vi "Main.vi"() -> ()   [LabVIEW 2015]
doc: "This Continuous Measurement sample project is based on the Queued Message Handler template.\n\nThe Event Handling Loop generates messages based on user interface actions.\n\nThe Message Handling Loop processes messages generated by the Event Handling Loop, or by other messages. There are also Acquisition and Logging message handling loop subVIs, and a chart updating loop."
uses:
  controls/Test Data.ctl
  controls/Tags.ctl
  controls/UI State.ctl
  controls/Flota.ctl
  support/Message Queue/Enqueue Message (Single).vi
  support/Message Queue/Enqueue Message (Array).vi
  <vilib>/Utility/error.llb/Error Cluster From Error Code.vi
  <vilib>/ErrorRing/Error Ring.xnode
  support/User Event - Stop/User Event - Stop.lvlib
  support/Message Queue/Message Queue.lvlib
panel:
  in  "Acq":T1
  in  "TAGs":T2
  out "Ultimo TEST":timestamp
  in  "Test":T3
  out "Reset del controlador":bool
  out "error":errorcluster
  in  "Developer commad":string
  out "Buffer Overflow":bool
  out "Buffer Underflow":bool
  in  "Calibration":bool
  out "Report":string
  in  "Exit":bool
  # "Opciones\n- Adquirir\n- STOP_WHD\n- Reset_Controlador"
  # "Misma función que introducir STOP_WHD\n en Developer command"
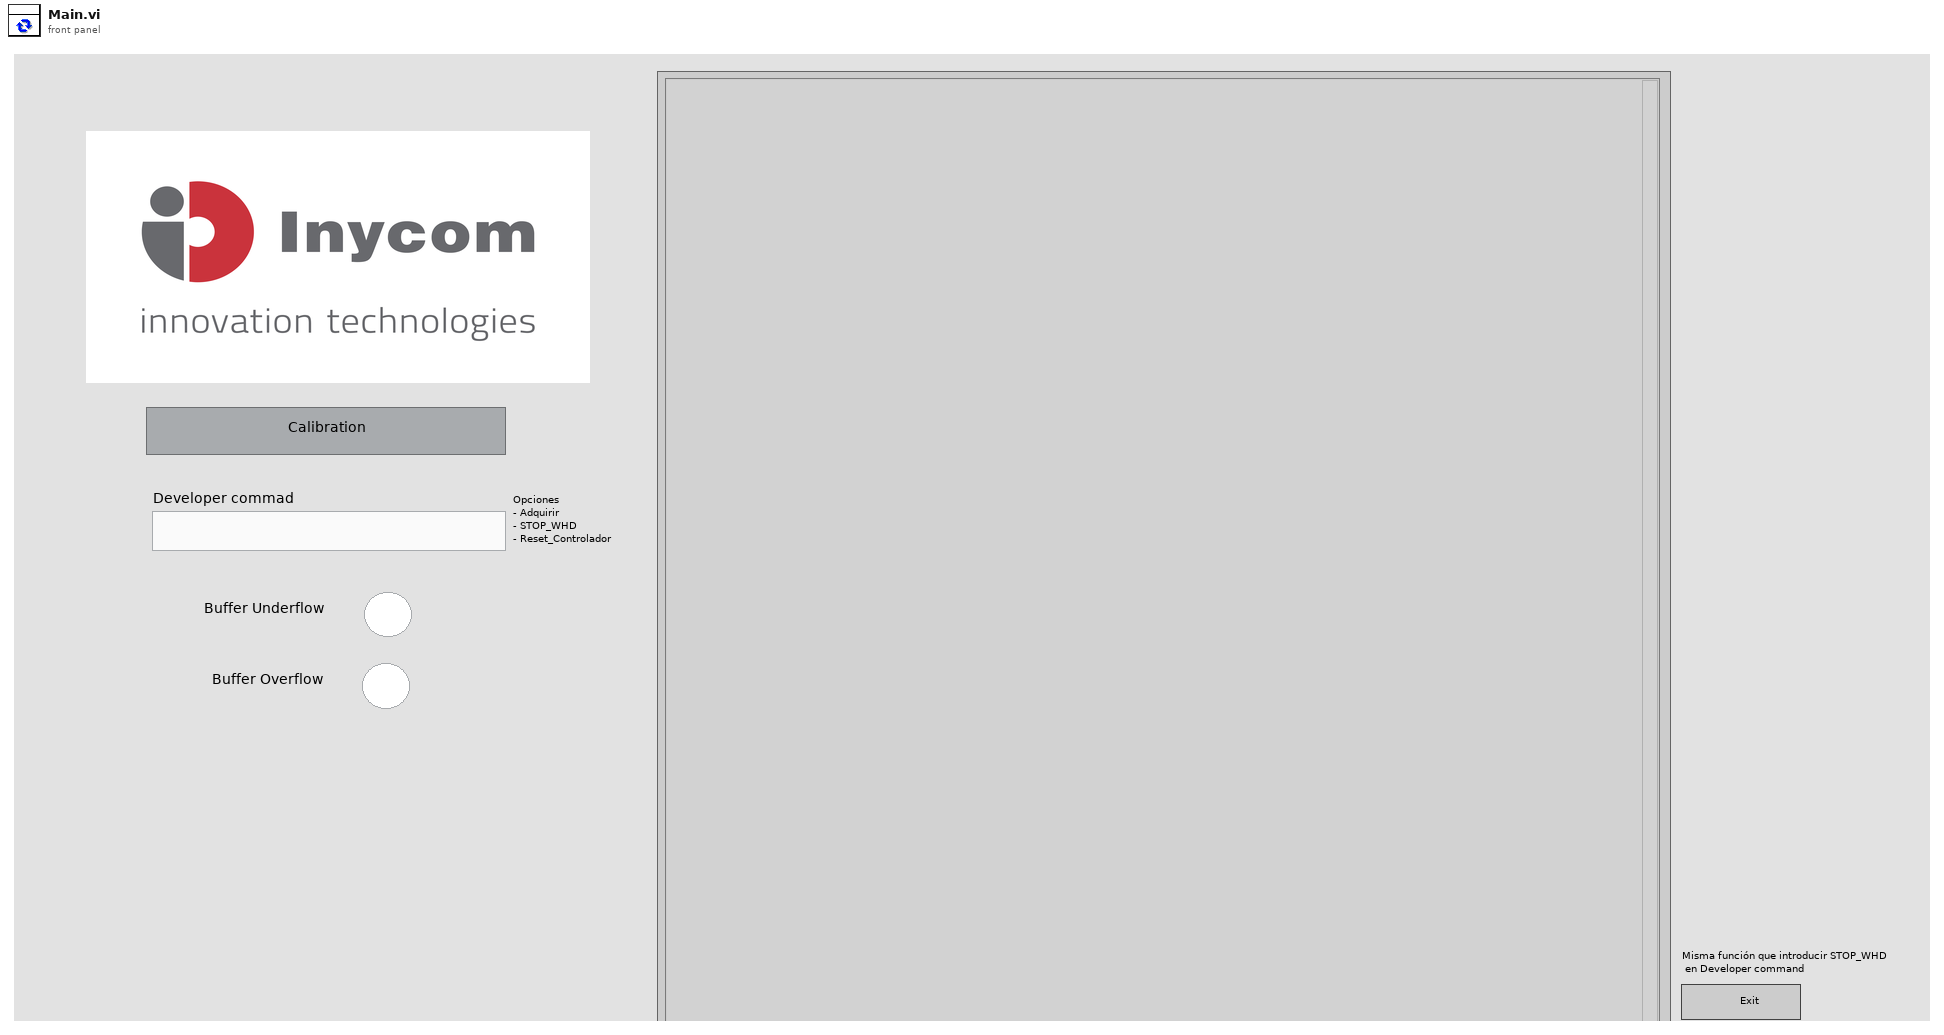
[diagram p1: front panel]
types:
  T1 = cluster{"FPGA error ":errorcluster, "data":dbl[], "Direccion 0?":bool, "File error ":errorcluster}
  T2 = typedef "Tags.ctl" = cluster{"TAGs":string[], "TAGs HEX":string[], "TAGs LR6":string[], "it-read-LR6":i32[], "it-LR6":i32}
  T3 = typedef "Test Data.ctl" = cluster{"DC OK":string, "Aviso temperatura":string, "Aviso no detección":string, "RuedaDetectada1?":bool, "RuedaDetectada2?":bool, "T fuera rango":bool, "Fallo Fotocelula":bool, "Timeout ruedas":bool, "Buffer Underflow":bool, "Buffer Overflow":bool, "Nº Ruedas 1":i32, "NºRuedas 2":i32, "Block Size":u32, "Time to Acquire Block (ms)":i32, "Ref file Data":refnum<file>[], "Number of elements":u32, "Tiempo de paso (s)":dbl}
  T4 = typedef "UI State.ctl" = enum16{"Idle", "Waiting_trigger", "Acquiring and Logging", "Calibration", "Waiting for Exit", "Waiting for Exit (Acq Stopped)", "Waiting for Exit (Log Stopped)", "Waiting for Stop", "Waiting for Stop (Acq Stopped)", "Waiting for Stop (Log Stopped)"}
  T5 = typedef "File paths.ctl" = cluster{"configuration":path, "confRFID":path, "LOG.txt":path, "Path LOG":path, "Path_data":path, "TAGS leidos":path, "configuracion flota":path, "flota":path, "Nombre de archivo":path[], "Folder calibration":path, "calibration log":path, "Reporting Procesamiento":path, "Error ejes":path, "Reporting Adquisición":path}
  T6 = cluster{"error IO":errorcluster, bool[], u32[], string[], dbl[]}
  T7 = typedef "Cfg_parameters.ctl" = cluster{"RFID NEM on?":bool, "RFID LR6 on?":bool, "Use Aura?":bool, "Leer config RFID NEM":bool, "Canal cero WS1?":bool, "Canal cero WS2 ":bool, "Digital?":bool, "Reset watchdog?":bool, "Able watchdog?":bool, "Borrar archivos\nadquisicion con error":bool, "AURA wheel test":bool, "Save calibration":bool, "Puerto RFID":u16, "Port LR6":u16, "timeout ms (60000)":i32, "bytes to read":i32, "DeviceAddress":u8, "IP RFID":string, "IP synchr":string, "LR6 IP address":string, "Parametros AuraWheel":string[], "Frecuencia de muestreo y módulo CRIO":T8, "Escaneos de la FIFO por canal":u32, "Frecuencia de muestreo (Hz)":dbl, "dt RMS":dbl, "Tiempo extra al detector de paso (s)":dbl, "Count(mSec)":u32, "Offset_rueda WS 1":fxp<+/-,24,-4>, "Offset_rueda WS 2":fxp<+/-,24,-4>, "Nº de acelerómetros":i32, "Nº inductivos":i32, "Max archivos":u32, "Bytes min libre":u32, "Bytes libre despues de borrar":u32, "Timeout ruedas":dbl, "Pattern amplitude (g)":dbl, "Pattern frequency (Hz)":dbl, "Tiempo de adquisicion\n":dbl, "Parámetros acelerómetros":dbl[], "Inicio pasada":timestamp, "Ultimo TEST":timestamp, "Report_AURA":string, "Temperatura (ºC)":dbl, "Direccion 0?":bool}
  T8 = typedef "nicrio_cRIO-9234_DataRatesRing2.ctl" = u8
  T9 = typedef "Message Queue.lvlib/All Message Queues.ctl" = cluster{"UI":refnum<queue>, "Acquisition and Logging":refnum<queue>, "RFID":refnum<queue>, "Processing":refnum<queue>, "Watchdog":refnum<queue>, "Calibration":refnum<queue>}
  T10 = typedef "Flota.ctl" = cluster{"Series_flota":string[], "Distancia de acelerómetros":dbl[], "Puntos medios de las ventanas":dbl[][], "Distancias generales":dbl[], "Tabla_flota":string[][]}
  T11 = cluster{"Distacias y medidas de dispositivos":bool, "Lectura_OK?":bool}
  T12 = cluster{"FPGA error ":errorcluster, "data":dbl[], "TAGs":string[], "Direccion 0?":bool}
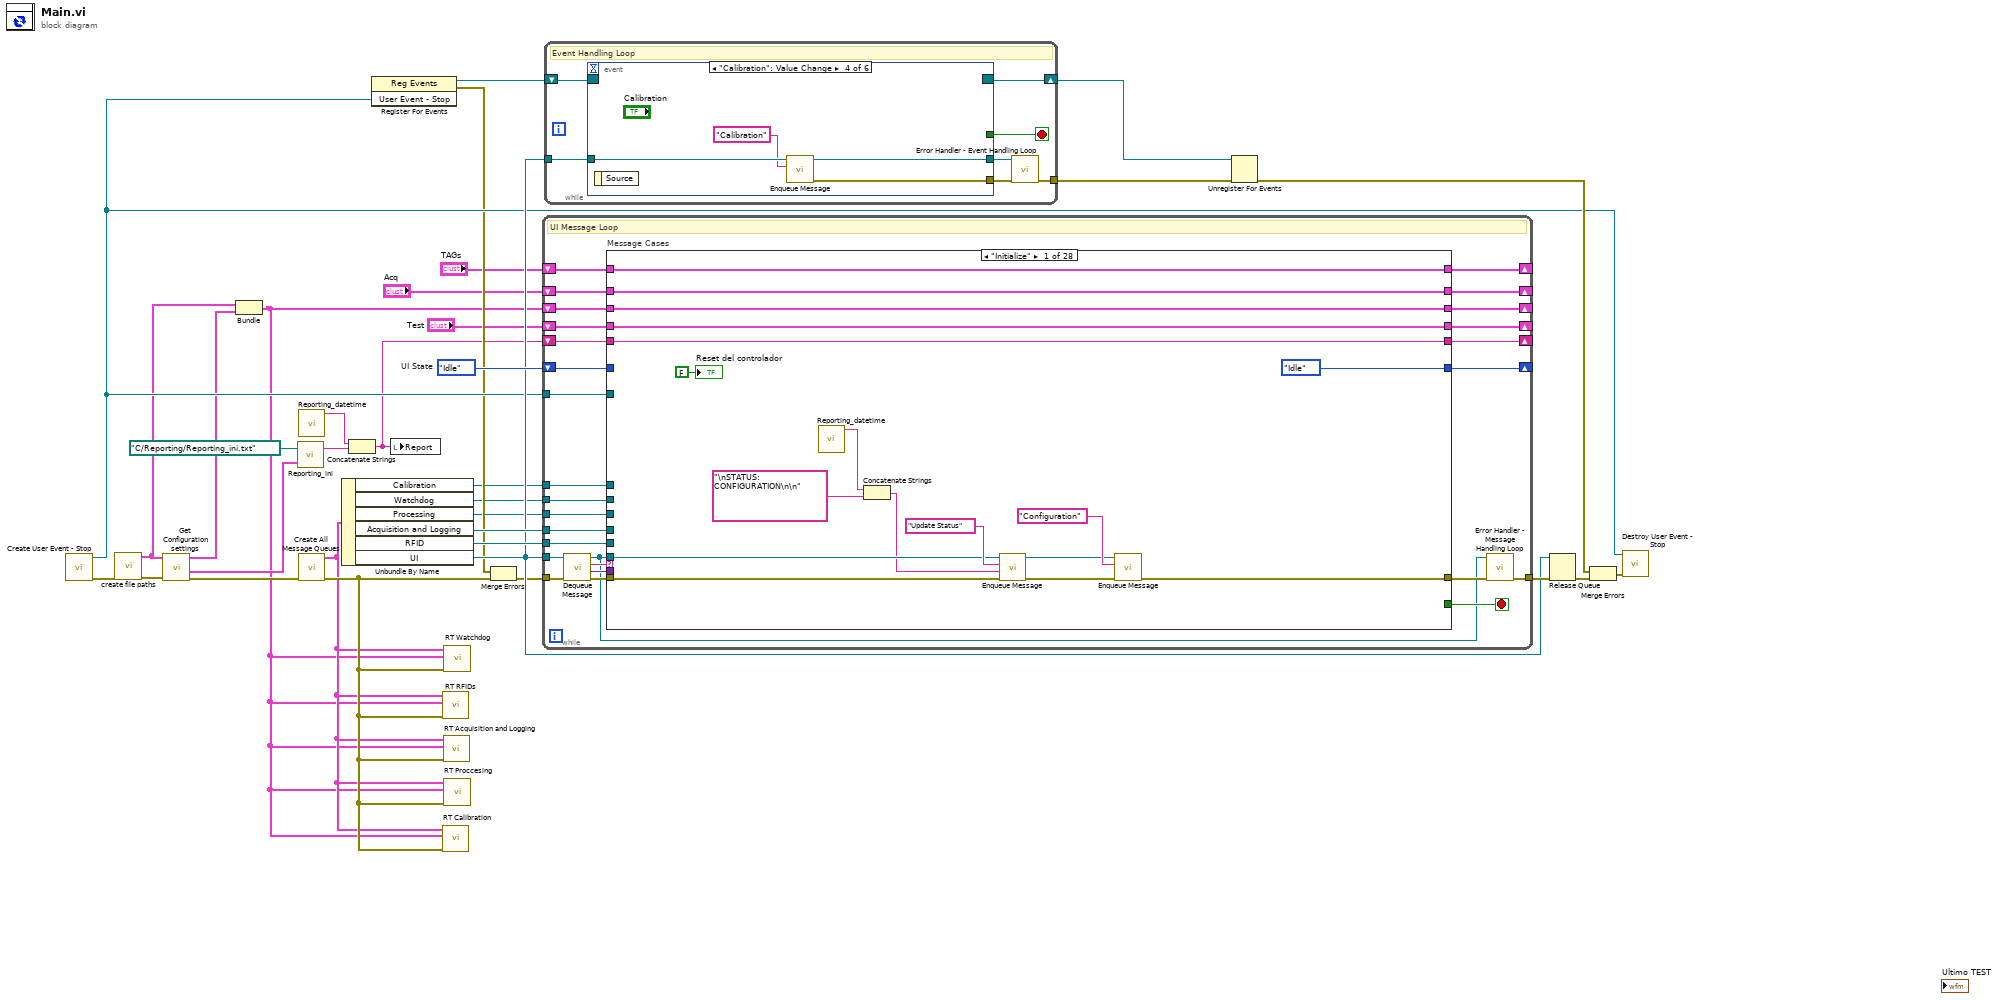
[diagram p0: block diagram]
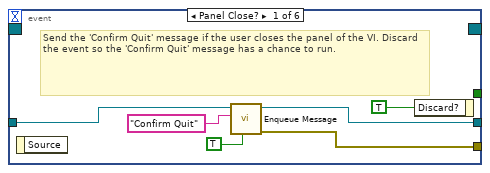
[diagram p2: hidden frame]
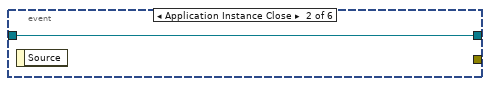
[diagram p3: hidden frame]
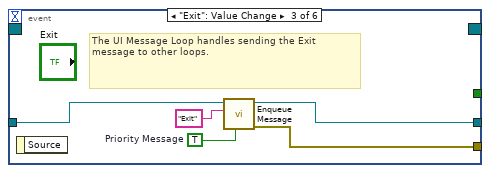
[diagram p4: hidden frame]
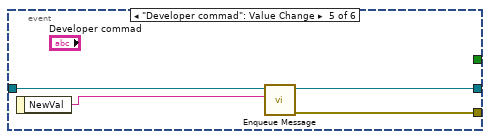
[diagram p5: hidden frame]
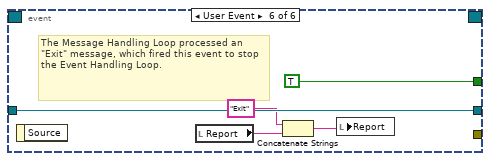
[diagram p6: hidden frame]
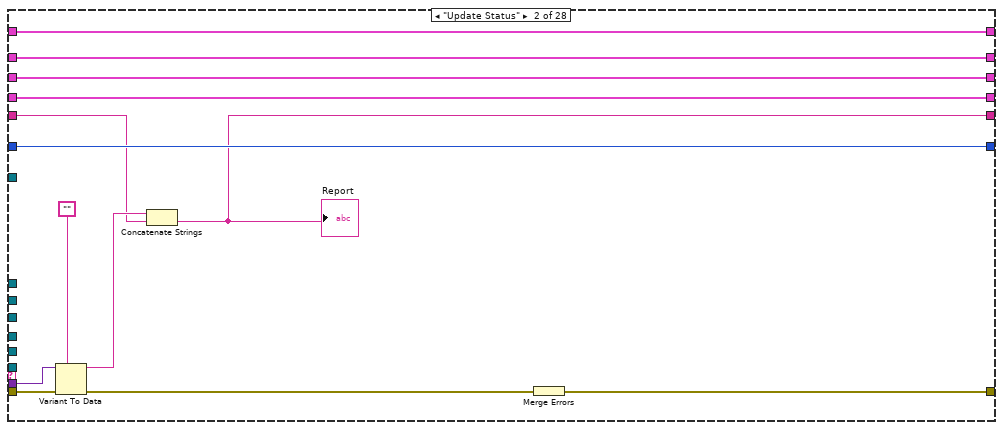
[diagram p7: hidden frame]
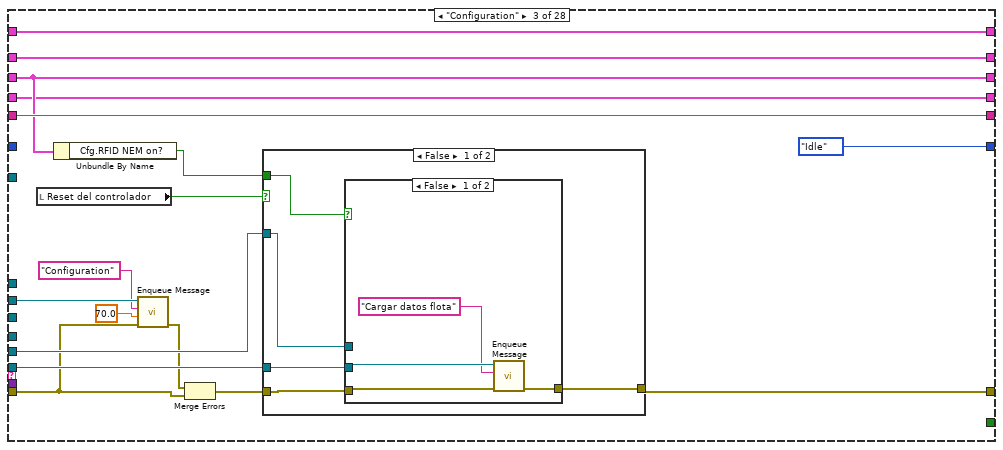
[diagram p8: hidden frame]
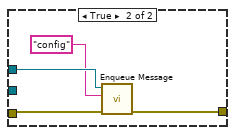
[diagram p9: hidden frame]
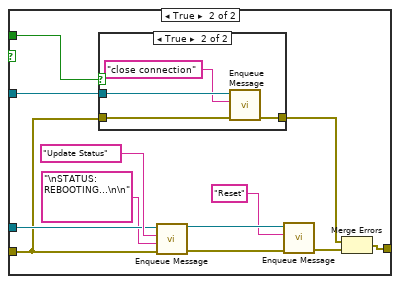
[diagram p10: hidden frame]
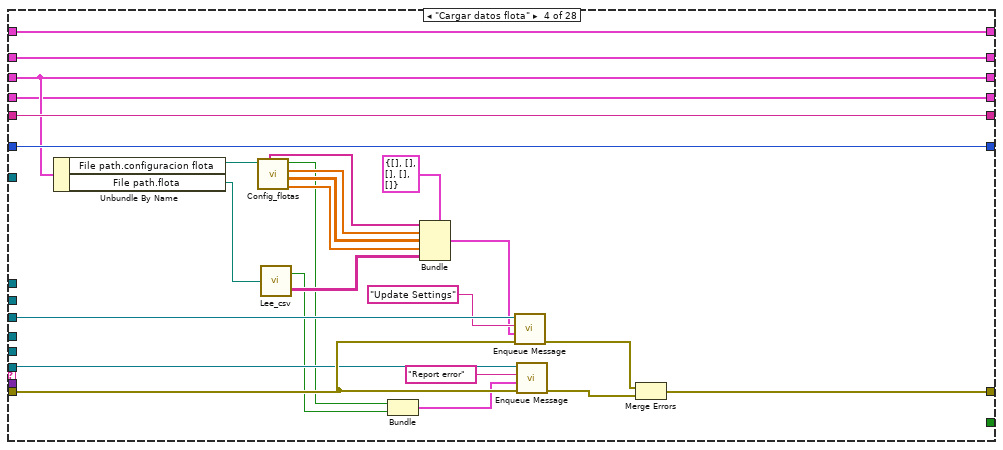
[diagram p12: hidden frame]
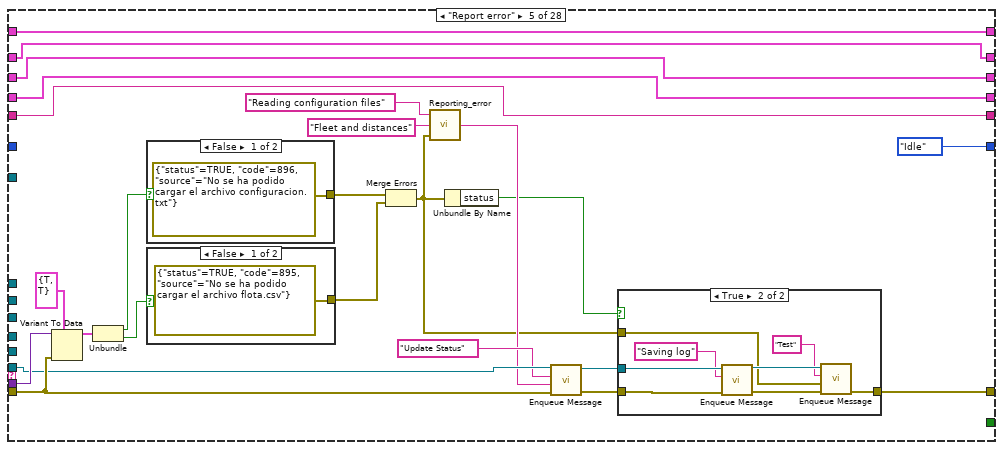
[diagram p13: hidden frame]
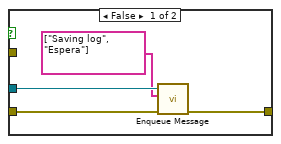
[diagram p14: hidden frame]
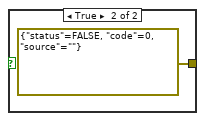
[diagram p15: hidden frame]
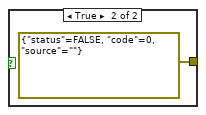
[diagram p16: hidden frame]
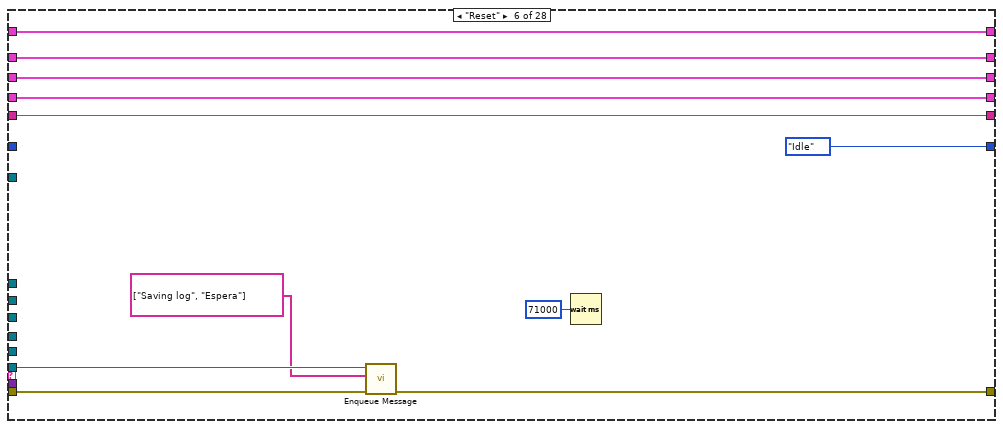
[diagram p17: hidden frame]
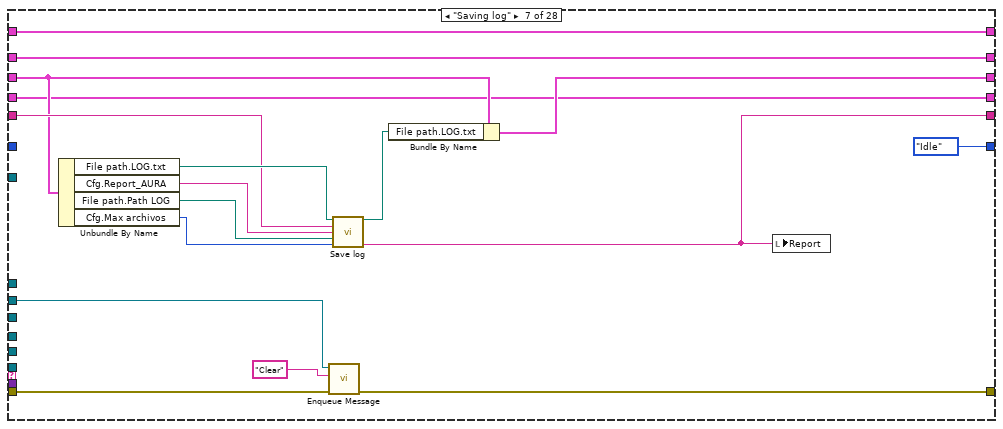
[diagram p18: hidden frame]
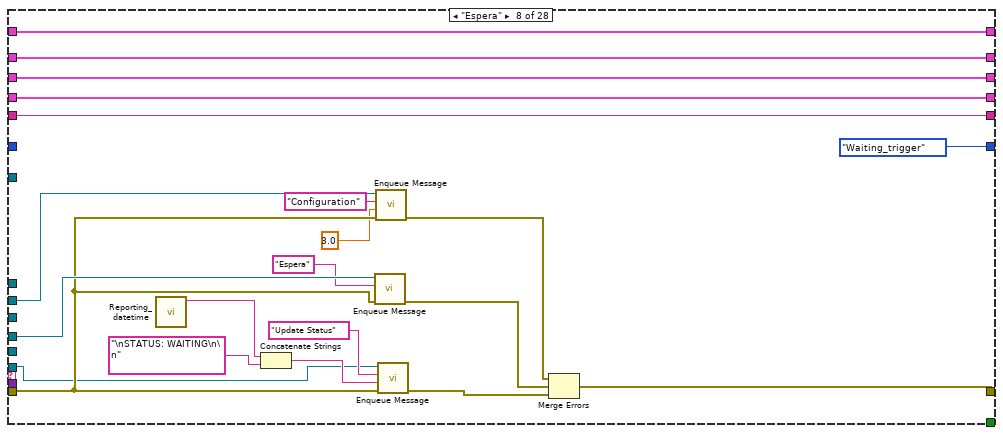
[diagram p19: hidden frame]
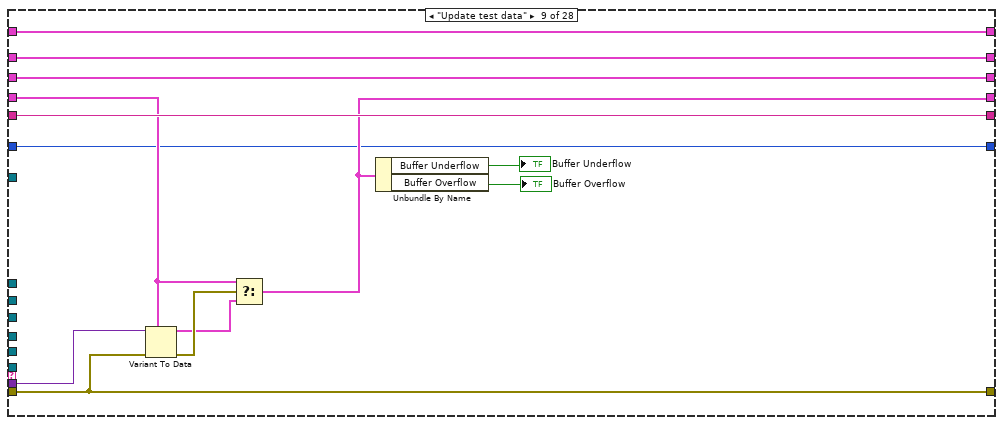
[diagram p20: hidden frame]
diagram:
  w27 = UI_State."Idle"  # UI State
  n1 = call "Create User Event - Stop.vi"() -> ("error out"=w13:errorcluster, "User Event - Stop"=w23:refnum<user-event>)  [unwired: 10 in]
  n2 = call "create file paths.vi"("error in"=w13) -> ("error out"=w12:errorcluster, "File path"=w11:T5)  [unwired: 9 in]
  n3 = call "Get Configuration settings.vi"("error in (no error)"=w12, "File path"=w11) -> ("error out"=w19:errorcluster, "output cluster"=w14:T6, "Cfg"=w10:T7)  [unwired: 5 in]
  n4 = Bundle("File path"=w11, "Cfg"=w10) -> (w2:cluster{"File path":T5, "Cfg ":T7})  [unwired: 1 in]
  n5 = call "Reporting_ini.vi"("Configuration cluster"=w14, "address repoting"=path "C:/Reporting/Reporting_ini.txt" ("file (use dialog)")) -> ("Reporting"=w17:string)  [unwired: 1 in]
  n6 = call "Reporting_datetime.vi"() -> ("String"=w16:string)  [unwired: 11 in]
  n7 = call "Create All Message Queues.vi"("error in (no error)"=w19) -> ("error out"=w4:errorcluster, "Message Queues out"=w3:T9)  [unwired: 9 in]
  n8 = Unbundle By Name(w3) -> ("Calibration"=w1:refnum<queue>, "Watchdog"=w8:refnum<queue>, "Processing"=w9:refnum<queue>, "Acquisition and Logging"=w29:refnum<queue>, "RFID"=w28:refnum<queue>, "UI"=w25:refnum<queue>)
  n9 = Concatenate Strings(w16, w17) -> (w15:string)
  n10 = register-events(w23) -> (reference out=w24:refnum<event-registration>, error out=w21:errorcluster)  [unwired: 2 in]
  n11 = local write "Report"(w15) -> ()
  n12 = call "RT RFIDs.vi"("error in (no error)"=w4, "info"=w2, "Message Queues in"=w3) -> ()  [unwired: 8 in, 1 out]
  n13 = call "RT Calibration.vi"("error in (no error)"=w4, "info"=w2, "Message Queues in"=w3) -> ()  [unwired: 8 in, 1 out]
  n14 = call "RT Acquisition and Logging.vi"("error in (no error)"=w4, "info"=w2, "Message Queues in"=w3) -> ()  [unwired: 8 in, 1 out]
  n15 = call "RT Watchdog.vi"("error in (no error)"=w4, "info"=w2, "Message Queues in"=w3) -> ()  [unwired: 8 in, 1 out]
  n16 = call "RT Proccesing.vi"("error in (no error)"=w4, "info"=w2, "Message Queues in"=w3) -> ()  [unwired: 8 in, 1 out]
  n17 = Merge Errors(w21, w4) -> (w22:errorcluster)
  n18 = while {
    tunnel: w25 -> [w54]
    tunnel: w23 -> [w59]
    shift-right: [w53] -> _
    shift-left: w2 -> [w52]
    tunnel: w29 -> [w51]
    tunnel: w28 -> [w50]
    shift-right: [w45] -> _
    shift-left: w27 -> [w46]
    tunnel: w22 -> [w58]
    tunnel: [w49] -> w33
    shift-right: [w43] -> _
    shift-left: w15 -> [w44]
    tunnel: w9 -> [w42]
    tunnel: w8 -> [w41]
    shift-right: [w39] -> _
    shift-left: "Test" -> [w40]
    shift-right: [w37] -> _
    shift-left: "TAGs" -> [w38]
    shift-right: [w35] -> _
    shift-left: "Acq" -> [w36]
    tunnel: w1 -> [w34]
    stop <- w60 stop-if-true
    # "UI Message Loop"
    n19 = call "Dequeue Message.vi"("error in (no error)"=w58, "Message Queue"=w54) -> ("error out"=w57:errorcluster, "Message Data"=w55:variant, "Message"=w56:string, "dup Message Queue"=w47:refnum<queue>)  [unwired: 6 in]
    n20 = case "Message Cases" shown="\"Initialize\"" w56 {
      selector: w56 -> [_ _ _ _ _ _ _ _ _ w271 _ _ _ _ _ _ _ _ _ _ _ _ _ _ _ _ _ w664]
      tunnel: w47 -> [w75 _ w102 w145 w175 w208 _ w236 _ _ w287 w300 _ w347 w379 w390 w438 w472 w491 w514 w541 w566 _ _ w609 _ _ _]
      tunnel: w57 -> [w74 w89 w96 w149 w176 w209 w222 w245 w260 w275 w286 w301 w320 w343 w365 w392 w439 w473 w492 w511 w527 w557 w582 w595 w608 w644 w658 _]
      tunnel: [w66 w90 w100 w148 w173 w210 w220 w244 w260 w275 w285 w299 w321 w339 w374 w391 w437 w471 w490 w508 w535 w559 w582 w597 w607 w648 w657 w663] -> w48
      tunnel: [_ _ _ _ _ _ _ _ _ _ _ _ _ _ _ _ _ _ _ _ _ _ _ _ _ TRUE _ _] -> w60
      tunnel: w55 -> [_ w88 _ _ w187 _ _ _ w261 _ _ _ _ _ w364 w402 w444 w479 w498 _ _ _ w580 w598 _ w642 _ _]
      tunnel: w59 -> [_ _ _ _ _ _ _ _ _ _ _ _ _ _ _ _ _ _ _ _ _ _ _ _ _ w649 _ _]
      tunnel: [w72 w83 w105 w161 w168 w214 w223 w252 w265 w274 w292 w303 w326 w350 w383 w387 w446 w482 w501 w519 w543 w576 w578 w601 w611 w647 w656 w666] -> w53
      tunnel: w52 -> [w72 w83 w105 w161 w168 w214 w225 w252 w265 w274 w292 w303 w326 w350 w383 w388 w446 w482 w501 w519 w543 w576 w579 w601 w611 w647 w656 w666]
      tunnel: w51 -> [_ _ _ _ _ _ _ w247 _ w272 _ w296 w319 _ _ _ w435 _ _ _ _ _ _ _ _ w640 _ _]
      tunnel: w50 -> [_ _ w101 _ _ _ _ _ _ _ _ _ _ w348 _ _ _ _ _ _ _ _ _ _ _ w646 _ _]
      tunnel: w46 -> [_ w85 _ w162 _ _ _ _ w253 w270 w290 w298 w324 _ _ _ _ w469 w488 _ _ w571 w585 w596 w610 _ w655 w665]
      tunnel: [UI_State."Idle" ("UI State") w85 UI_State."Idle" ("UI State") w162 UI_State."Idle" ("UI State") UI_State."Idle" ("UI State") UI_State."Idle" ("UI State") UI_State."Waiting_trigger" ("UI State") w253 w269 w290 w297 w323 UI_State."Acquiring and Logging" ("UI State") UI_State."Idle" ("UI State") UI_State."Idle" ("UI State") UI_State."Idle" ("UI State") UI_State."Waiting for Stop (Acq Stopped)" ("UI State") UI_State."Waiting for Stop (Acq Stopped)" ("UI State") UI_State."Idle" ("UI State") UI_State."Idle" ("UI State") w571 w585 w596 w606 UI_State."Idle" ("UI State") w655 w665] -> w45
      tunnel: w44 -> [w73 w81 w106 w163 w178 w211 w229 w237 w264 w273 w291 w302 w325 w335 w367 w393 w433 w477 w494 w525 w546 w572 w586 w594 w605 w641 w654 w662]
      tunnel: [w73 w84 w106 w163 w178 w211 w215 w237 w264 w273 w291 w302 w325 w335 w367 w393 w433 w477 w494 w525 w546 w572 w586 w594 w605 w641 w654 w662] -> w43
      tunnel: w42 -> [_ _ _ w152 _ _ _ _ _ _ _ _ _ _ _ _ _ _ _ _ _ w558 _ _ _ w639 _ _]
      tunnel: w41 -> [_ _ w99 _ _ _ w221 w246 _ _ _ _ _ w344 w375 w384 _ _ _ _ w534 w563 _ _ _ w638 _ _]
      tunnel: w40 -> [w63 w80 w93 w140 w169 w206 w218 w234 w259 w268 w283 w295 w322 w336 w368 w389 w434 w478 w495 w526 w542 w573 w587 w592 w604 w636 w653 w661]
      tunnel: [w63 w80 w93 w140 w169 w206 w218 w234 w258 w268 w283 w295 w322 w336 w368 w389 w434 w478 w495 w526 w542 w573 w587 w592 w604 w636 w653 w661] -> w39
      tunnel: w38 -> [w62 w79 w92 w139 w167 w205 w217 w233 w255 w267 w282 w294 w318 w338 w361 w386 w431 w476 w497 w522 w544 w575 w589 w591 w603 w635 w652 w660]
      tunnel: [w62 w79 w92 w139 w167 w205 w217 w233 w255 w267 w282 w294 w318 w338 w361 w386 w431 w476 w496 w522 w544 w575 w589 w591 w603 w635 w652 w660] -> w37
      tunnel: w36 -> [w61 w78 w91 w138 w166 w204 w216 w232 w254 w266 w281 w293 w317 w337 w360 w385 w430 w475 w493 w523 w532 w574 w588 w590 w602 w634 w651 w659]
      tunnel: [w61 w78 w91 w138 w166 w204 w216 w232 w254 w266 w281 w293 w317 w337 w360 w385 w430 w474 w493 w523 w532 w574 w588 w590 w602 w634 w651 w659] -> w35
      tunnel: w34 -> [_ _ _ _ _ _ _ _ _ _ _ _ _ _ _ _ _ _ _ _ _ _ _ _ _ w633 _ _]
      frame "Initialize" {
        # "Initialize - Get configuration settings, then message the UI to initialize, and broadcast the settings to the other message loops."
        n21 = call "Reporting_datetime.vi"() -> ("String"=w70:string)  [unwired: 11 in]
        n22 = Concatenate Strings(w70, "\nSTATUS: CONFIGURATION\n\n") -> (w69:string)
        n23 = call-poly "Enqueue Message.vi"("error in (no error)"=w74, "Message Data"=w69, "Message"="Update Status", "Message Queue"=w75) -> ("error out"=w67:errorcluster, "dup Message Queue"=w65:refnum<queue>)  [unwired: 6 in]
        n24 = call-poly "Enqueue Message.vi"("error in (no error)"=w67, "Message"="Configuration", "Message Queue"=w65) -> ("error out"=w66:errorcluster)  [unwired: 7 in, 1 out]
        "Reset del controlador" <- FALSE ("Reset del controlador")
      }
      frame "Update Status" {
        # "Update Status - Convert the message data to a string to display in the Status indicator."
        n25 = Variant To Data(error in=w89, type="", Variant=w88) -> (data=w82:string, error out=w86:errorcluster)
        n26 = Concatenate Strings(w82, w81) -> (w84:string)
        "Report" <- w84
        n27 = Merge Errors(w86) -> (w90:errorcluster)
      }
      frame "Configuration" {
        n28 = local read "Reset del controlador"() -> (w104:bool)
        n29 = Unbundle By Name(w105) -> ("Cfg.RFID NEM on?"=w103:bool)
        n30 = call-poly "Enqueue Message.vi"("error in (no error)"=w96, "Message Data"=70.0, "Message"="Configuration", "Message Queue"=w99) -> ("error out"=w95:errorcluster)  [unwired: 6 in, 1 out]
        n31 = Merge Errors(w95, w96) -> (w97:errorcluster)
        n32 = case shown="False" w104 {
          tunnel: w103 -> [w112 w124]
          tunnel: w97 -> [w111 w126]
          tunnel: w102 -> [w110 w131]
          tunnel: w101 -> [w109 w125]
          tunnel: [w108 w121] -> w100
          frame False {
            n33 = case shown="False" w112 {
              tunnel: w111 -> [w116 w119]
              tunnel: w110 -> [w114 _]
              tunnel: w109 -> [_ w118]
              tunnel: [w115 w120] -> w108
              frame False {
                n34 = call-poly "Enqueue Message.vi"("error in (no error)"=w116, "Message"="Cargar datos flota", "Message Queue"=w114) -> ("error out"=w115:errorcluster)  [unwired: 7 in, 1 out]
              }
              frame True {
                n35 = call-poly "Enqueue Message.vi"("error in (no error)"=w119, "Message"="config", "Message Queue"=w118) -> ("error out"=w120:errorcluster)  [unwired: 7 in, 1 out]
              }
            }
          }
          frame True {
            n36 = case shown="True" w124 {
              tunnel: w126 -> [w133 w137]
              tunnel: w125 -> [_ w136]
              tunnel: [w133 w134] -> w122
              frame False {
              }
              frame True {
                n37 = call-poly "Enqueue Message.vi"("error in (no error)"=w137, "Message"="close connection", "Message Queue"=w136) -> ("error out"=w134:errorcluster)  [unwired: 7 in, 1 out]
              }
            }
            n38 = call-poly "Enqueue Message.vi"("error in (no error)"=w126, "Message Data"="\nSTATUS: REBOOTING...\n\n", "Message"="Update Status", "Message Queue"=w131) -> ("error out"=w128:errorcluster, "dup Message Queue"=w129:refnum<queue>)  [unwired: 6 in]
            n39 = call-poly "Enqueue Message.vi"("error in (no error)"=w128, "Message"="Reset", "Message Queue"=w129) -> ("error out"=w123:errorcluster)  [unwired: 7 in, 1 out]
            n40 = Merge Errors(w122, w123) -> (w121:errorcluster)
          }
        }
      }
      frame "Cargar datos flota" {
        n41 = Unbundle By Name(w161) -> ("File path.configuracion flota"=w160:path, "File path.flota"=w153:path)
        n42 = call "Config_flotas.vi"("file path (dialog if empty)"=w160) -> ("Distancias generales"=w155:dbl[], "Puntos medios de las ventanas"=w156:dbl[][], "Distancia de acelerómetros"=w157:dbl[], "Distacias y medidas de dispositivos"=w142:bool, "Series_flota"=w159:string[])  [unwired: 3 in]
        n43 = call "Lee_csv.vi"("Path"=w153) -> ("Tabla_flota"=w154:string[][], "Lectura_OK?"=w143:bool)
        n44 = Bundle("Distacias y medidas de dispositivos"=w142, "Lectura_OK?"=w143) -> (w144:T11)  [unwired: 1 in]
        n45 = Bundle(cluster=T10 {"Series_flota"=[], "Distancia de acelerómetros"=[], "Puntos medios de las ventanas"=[], "Distancias generales"=[], "Tabla_flota"=[]} ("Flota"), "Series_flota"=w159, "Distancia de acelerómetros"=w157, "Puntos medios de las ventanas"=w156, "Distancias generales"=w155, "Tabla_flota"=w154) -> (w150:T10)
        n46 = call-poly "Enqueue Message.vi"("error in (no error)"=w149, "Message Data"=w150, "Message"="Update Settings", "Message Queue"=w152) -> ("error out"=w147:errorcluster)  [unwired: 6 in, 1 out]
        n47 = call-poly "Enqueue Message.vi"("error in (no error)"=w149, "Message Data"=w144, "Message"="Report error", "Message Queue"=w145) -> ("error out"=w146:errorcluster)  [unwired: 6 in, 1 out]
        n48 = Merge Errors(w147, w146) -> (w148:errorcluster)
      }
      frame "Report error" {
        n49 = Variant To Data(error in=w176, type=cluster{bool, bool} {TRUE, TRUE}, Variant=w187) -> (data=w185:cluster{bool, bool})  [unwired: 1 out]
        n50 = Unbundle(w185) -> (w180:bool, w179:bool)
        n51 = case shown="False" w180 {
          tunnel: [errorcluster {"status"=TRUE, "code"=896, "source"="No se ha podido cargar el archivo configuracion.txt"} ("error out") errorcluster {"status"=FALSE, "code"=0, "source"=""} ("error out")] -> w184
          frame False {
          }
          frame True {
          }
        }
        n52 = case shown="False" w179 {
          tunnel: [errorcluster {"status"=TRUE, "code"=895, "source"="No se ha podido cargar el archivo flota.csv"} ("error out") errorcluster {"status"=FALSE, "code"=0, "source"=""} ("error out")] -> w183
          frame False {
          }
          frame True {
          }
        }
        n53 = Merge Errors(w184, w183) -> (w164:errorcluster)
        n54 = call "Reporting_error.vi"("error out 2"=w164, "Concept explanation"="Fleet and distances", "Concept"="Reading configuration files") -> ("Reporting"=w170:string)
        n55 = Unbundle By Name(w164) -> ("status"=w165:bool)
        n56 = call-poly "Enqueue Message.vi"("error in (no error)"=w176, "Message Data"=w170, "Message"="Update Status", "Message Queue"=w175) -> ("error out"=w172:errorcluster, "dup Message Queue"=w171:refnum<queue>)  [unwired: 6 in]
        n57 = case shown="True" w165 {
          tunnel: [w190 w195] -> w173
          tunnel: w172 -> [w191 w199]
          tunnel: w171 -> [w189 w198]
          tunnel: w164 -> [_ w193]
          frame False {
            n58 = call-poly "Enqueue Message.vi"("error in (no error)"=w191, "Message Array"=string[] ["Saving log", "Espera"], "Message Queue"=w189) -> ("error out"=w190:errorcluster)  [unwired: 7 in, 1 out]
          }
          frame True {
            n59 = call-poly "Enqueue Message.vi"("error in (no error)"=w199, "Message"="Saving log", "Message Queue"=w198) -> ("error out"=w196:errorcluster, "dup Message Queue"=w197:refnum<queue>)  [unwired: 7 in]
            n60 = call-poly "Enqueue Message.vi"("error in (no error)"=w196, "Message Data"=w193, "Message"="Test", "Message Queue"=w197) -> ("error out"=w195:errorcluster)  [unwired: 6 in, 1 out]
          }
        }
      }
      frame "Reset" {
        n61 = call-poly "Enqueue Message.vi"("error in (no error)"=w209, "Message Array"=string[] ["Saving log", "Espera"], "Message Queue"=w208) -> ("error out"=w210:errorcluster)  [unwired: 7 in, 1 out]
        n62 = Wait (ms)(milliseconds to wait=u32 71000) -> ()  [unwired: 1 out]
      }
      frame "Saving log" {
        n63 = Unbundle By Name(w225) -> ("File path.LOG.txt"=w230:path, "Cfg.Report_AURA"=w228:string, "File path.Path LOG"=w227:path, "Cfg.Max archivos"=w226:u32)
        n64 = call-poly "Enqueue Message.vi"("error in (no error)"=w222, "Message"="Clear", "Message Queue"=w221) -> ("error out"=w220:errorcluster)  [unwired: 7 in, 1 out]
        n65 = call "Save log.vi"("Path"=w230, "Report in"=w229, "Report AURA"=w228, "Path Carpeta"=w227, "Nº Archivos Max"=w226) -> ("path"=w224:path, "Report out"=w215:string)  [unwired: 9 in]
        n66 = Bundle By Name(cluster=w225, "File path.LOG.txt"=w224) -> (w223:cluster{"File path":T5, "Cfg ":T7})
        n67 = local write "Report"(w215) -> ()
      }
      frame "Espera" {
        n68 = call "Reporting_datetime.vi"() -> ("String"=w248:string)  [unwired: 11 in]
        n69 = Concatenate Strings(w248, "\nSTATUS: WAITING\n\n") -> (w250:string)
        n70 = call-poly "Enqueue Message.vi"("error in (no error)"=w245, "Message"="Espera", "Message Queue"=w247) -> ("error out"=w242:errorcluster)  [unwired: 7 in, 1 out]
        n71 = call-poly "Enqueue Message.vi"("error in (no error)"=w245, "Message Data"=3.0, "Message"="Configuration", "Message Queue"=w246) -> ("error out"=w243:errorcluster)  [unwired: 6 in, 1 out]
        n72 = call-poly "Enqueue Message.vi"("error in (no error)"=w245, "Message Data"=w250, "Message"="Update Status", "Message Queue"=w236) -> ("error out"=w241:errorcluster)  [unwired: 6 in, 1 out]
        n73 = Merge Errors(w243, w242, w241) -> (w244:errorcluster)
      }
      frame "Update test data" {
        n74 = Variant To Data(error in=w260, type=w259, Variant=w261) -> (data=w262:T3, error out=w263:errorcluster)
        n75 = Select(t=w259, s=w263, f=w262) -> (s? t:f=w258:T3)
        n76 = Unbundle By Name(w258) -> ("Buffer Underflow"=→"Buffer Underflow":bool, "Buffer Overflow"=→"Buffer Overflow":bool)
      }
      frame "Adquirir" {
        n77 = case shown="\"Waiting_trigger\"" w270 {
          selector: w270 -> [w276 _]
          tunnel: w272 -> [_ w280]
          tunnel: w271 -> [_ w279]
          tunnel: [w276 UI_State."Idle" ("UI State")] -> w269
          frame "Idle", Default {
          }
          frame "Waiting_trigger" {
            n78 = local write "Developer commad"("" ("Developer commad")) -> ()
            n79 = call-poly "Enqueue Message.vi"("Message"=w279, "Message Queue"=w280) -> ()  [unwired: 8 in, 2 out]
          }
        }
      }
      frame "STOP_WHD" {
        w288 = TRUE  # Priority Message
        n80 = local write "Developer commad"("" ("Developer commad")) -> ()
        n81 = call-poly "Enqueue Message.vi"("Priority Message? (F)"=w288, "error in (no error)"=w286, "Message"="Exit", "Message Queue"=w287) -> ("error out"=w285:errorcluster)  [unwired: 6 in, 1 out]
      }
      frame "Reset_Controlador" {
        n82 = case shown="\"Waiting_trigger\"" w298 {
          selector: w298 -> [w304 _]
          tunnel: w301 -> [w305 w307]
          tunnel: w300 -> [_ w315]
          tunnel: [w305 w310] -> w299
          tunnel: [w304 UI_State."Idle" ("UI State")] -> w297
          tunnel: w296 -> [_ w308]
          frame "Idle", Default {
          }
          frame "Waiting_trigger" {
            n83 = local write "Reset del controlador"(TRUE ("Reset del controlador")) -> ()
            n84 = local write "Developer commad"("" ("Developer commad")) -> ()
            n85 = call-poly "Enqueue Message.vi"("error in (no error)"=w307, "Message"="Reset", "Message Queue"=w308) -> ("error out"=w309:errorcluster)  [unwired: 7 in, 1 out]
            n86 = call-poly "Enqueue Message.vi"("error in (no error)"=w307, "Message"="Configuration", "Message Queue"=w315) -> ("error out"=w311:errorcluster)  [unwired: 7 in, 1 out]
            n87 = Merge Errors(w309, w311) -> (w310:errorcluster)
          }
        }
      }
      frame "Calibration" {
        n88 = case shown="\"Waiting_trigger\"" w324 {
          selector: w324 -> [w328 _]
          tunnel: [w328 UI_State."Calibration" ("UI State")] -> w323
          tunnel: [w327 w332] -> w321
          tunnel: w320 -> [w327 w331]
          tunnel: w319 -> [_ w330]
          frame "Idle", Default {
          }
          frame "Waiting_trigger" {
            n89 = call-poly "Enqueue Message.vi"("error in (no error)"=w331, "Message"="Calibration", "Message Queue"=w330) -> ("error out"=w332:errorcluster)  [unwired: 7 in, 1 out]
          }
        }
      }
      frame "Acquisition" {
        n90 = Unbundle By Name(w350) -> ("Cfg.RFID LR6 on?"=w349:bool)
        n91 = call "Reporting_datetime.vi"() -> ("String"=w353:string)  [unwired: 11 in]
        n92 = case shown="True" w349 {
          tunnel: w348 -> [_ w359]
          tunnel: w343 -> [w355 w357]
          tunnel: [w355 w356] -> w340
          frame False {
          }
          frame True {
            n93 = call-poly "Enqueue Message.vi"("error in (no error)"=w357, "Message"="Start", "Message Queue"=w359) -> ("error out"=w356:errorcluster)  [unwired: 7 in, 1 out]
          }
        }
        n94 = Concatenate Strings(w353, "\nSTATUS: ACQUISITION\nTrain is passing\n\n") -> (w354:string)
        n95 = call-poly "Enqueue Message.vi"("error in (no error)"=w343, "Message Data"=200.0, "Message"="Configuration", "Message Queue"=w344) -> ("error out"=w341:errorcluster)  [unwired: 6 in, 1 out]
        n96 = call-poly "Enqueue Message.vi"("error in (no error)"=w343, "Message Data"=w354, "Message"="Update Status", "Message Queue"=w347) -> ("error out"=w342:errorcluster)  [unwired: 6 in, 1 out]
        n97 = Merge Errors(w340, w341, w342) -> (w339:errorcluster)
      }
      frame "Test" {
        n98 = call "Reporting_datetime.vi"() -> ("String"=w382:string)  [unwired: 11 in]
        n99 = Variant To Data(error in=w365, type=errorcluster {"status"=FALSE, "code"=0, "source"=""} ("error constant"), Variant=w364) -> (data=w362:errorcluster)  [unwired: 1 out]
        n100 = Concatenate Strings(w382, "\nSTATUS: ERROR TEST\n\n") -> (w378:string)
        n101 = call-poly "Enqueue Message.vi"("error in (no error)"=w365, "Message Data"=200.0, "Message"="Configuration", "Message Queue"=w375) -> ("error out"=w373:errorcluster)  [unwired: 6 in, 1 out]
        n102 = call-poly "Enqueue Message.vi"("error in (no error)"=w365, "Message Data"=w378, "Message"="Update Status", "Message Queue"=w379) -> ("error out"=w372:errorcluster, "dup Message Queue"=w370:refnum<queue>)  [unwired: 6 in]
        n103 = call-poly "Enqueue Message.vi"("error in (no error)"=w372, "Message Data"=w362, "Message"="Test_log", "Message Queue"=w370) -> ("error out"=w371:errorcluster)  [unwired: 6 in, 1 out]
        n104 = Merge Errors(w373, w371) -> (w374:errorcluster)
      }
      frame "Test_log" {
        n105 = Unbundle By Name(w388) -> ("Cfg.Ultimo TEST"=w396:timestamp)
        n106 = Get Date/Time In Seconds() -> (seconds since 1Jan1904=w401:timestamp)
        n107 = To Double Precision Float(number=w401) -> (double precision float=w400:dbl)
        n108 = Variant To Data(error in=w392, type=errorcluster {"status"=FALSE, "code"=0, "source"=""} ("error constant"), Variant=w402) -> (data=w394:errorcluster)  [unwired: 1 out]
        n109 = Subtract(x=w400, y=3600.0) -> (x-y=w399:dbl)
        n110 = To Time Stamp(1:w399) -> (0:w398:timestamp)
        n111 = In Range and Coerce(upper limit=w401, x=w396, lower limit=w398) -> (In Range?=w395:bool)  [unwired: 1 out]
        n112 = case shown="True" w395 {
          tunnel: w389 -> [w414 _]
          tunnel: w394 -> [w406 _]
          tunnel: w392 -> [w417 w425]
          tunnel: [w409 w424] -> w391
          tunnel: w390 -> [w419 w427]
          tunnel: w388 -> [w413 w429]
          tunnel: [w411 w429] -> w387
          tunnel: w384 -> [_ w421]
          frame False {
            n113 = call "Test_save log.vi"("error in (no error)"=w406, "Test"=w414) -> ("Report"=w405:string)  [unwired: 9 in]
            n114 = Get Date/Time In Seconds() -> (seconds since 1Jan1904=w412:timestamp)
            n115 = Bundle By Name(cluster=w413, "Cfg.Ultimo TEST"=w412, "Cfg.Report_AURA"=w405) -> (w411:cluster{"File path":T5, "Cfg ":T7})
            n116 = call-poly "Enqueue Message.vi"("error in (no error)"=w417, "Message Data"=w405, "Message"="Update Status", "Message Queue"=w419) -> ("error out"=w418:errorcluster, "dup Message Queue"=w416:refnum<queue>)  [unwired: 6 in]
            n117 = call-poly "Enqueue Message.vi"("error in (no error)"=w418, "Message"="Saving log", "Message Queue"=w416) -> ("error out"=w410:errorcluster, "dup Message Queue"=w408:refnum<queue>)  [unwired: 7 in]
            n118 = call-poly "Enqueue Message.vi"("error in (no error)"=w410, "Message Data"=w406, "Message"="Exit Test", "Message Queue"=w408) -> ("error out"=w409:errorcluster)  [unwired: 6 in, 1 out]
          }
          frame True {
            n119 = call-poly "Enqueue Message.vi"("error in (no error)"=w425, "Message"="Clear", "Message Queue"=w421) -> ("error out"=w423:errorcluster)  [unwired: 7 in, 1 out]
            n120 = call-poly "Enqueue Message.vi"("error in (no error)"=w425, "Message Data"=w425, "Message"="Exit Test", "Message Queue"=w427) -> ("error out"=w422:errorcluster)  [unwired: 6 in, 1 out]
            n121 = Merge Errors(w423, w422) -> (w424:errorcluster)
          }
        }
      }
      frame "Exit Test" {
        n122 = Variant To Data(error in=w439, type=errorcluster {"status"=FALSE, "code"=0, "source"=""} ("error constant"), Variant=w444) -> (data=w443:errorcluster)  [unwired: 1 out]
        n123 = Unbundle By Name(w434) -> ("T fuera rango"=w436:bool, "Fallo Fotocelula"=w442:bool)
        n124 = Unbundle By Name(w443) -> ("status"=w441:bool)
        n125 = Compound Arithmetic op=OR(w442, w441) -> (w440:bool)
        n126 = local write "Reset del controlador"(w440) -> ()
        n127 = case shown="False" w440 {
          tunnel: w439 -> [w450 w468]
          tunnel: w438 -> [w449 w466]
          tunnel: [w448 w467] -> w437
          tunnel: w436 -> [w451 _]
          tunnel: w435 -> [w447 _]
          frame False {
            n128 = case shown="True" w451 {
              tunnel: w450 -> [w455 w456]
              tunnel: w449 -> [w452 w462]
              tunnel: [w454 w461] -> w448
              tunnel: w447 -> [_ w458]
              frame False {
                n129 = call-poly "Enqueue Message.vi"("error in (no error)"=w455, "Message"="Espera", "Message Queue"=w452) -> ("error out"=w454:errorcluster)  [unwired: 7 in, 1 out]
              }
              frame True {
                n130 = call-poly "Enqueue Message.vi"("error in (no error)"=w456, "Message"="UPS", "Message Queue"=w458) -> ("error out"=w459:errorcluster)  [unwired: 7 in, 1 out]
                n131 = call-poly "Enqueue Message.vi"("error in (no error)"=w456, "Message Data"="FAIL DC POWER\nUPS State", "Message"="Update Status", "Message Queue"=w462) -> ("error out"=w460:errorcluster)  [unwired: 6 in, 1 out]
                n132 = Merge Errors(w459, w460) -> (w461:errorcluster)
              }
            }
          }
          frame True {
            n133 = call-poly "Enqueue Message.vi"("error in (no error)"=w468, "Message"="Configuration", "Message Queue"=w466) -> ("error out"=w467:errorcluster)  [unwired: 7 in, 1 out]
          }
        }
      }
      frame "Update Acq data" {
        n134 = Variant To Data(error in=w473, type=w475, Variant=w479) -> (data=w480:T1, error out=w481:errorcluster)
        n135 = Select(t=w475, s=w481, f=w480) -> (s? t:f=w474:T1)
        n136 = case shown="\"Waiting for Stop (Acq Stopped)\"" w469 {
          tunnel: w473 -> [w483 w487]
          tunnel: w472 -> [_ w486]
          tunnel: [w483 w485] -> w471
          frame "Idle", Default {
          }
          frame "Waiting for Stop (Acq Stopped)" {
            n137 = call-poly "Enqueue Message.vi"("error in (no error)"=w487, "Message"="Acq report", "Message Queue"=w486) -> ("error out"=w485:errorcluster)  [unwired: 7 in, 1 out]
          }
        }
      }
      frame "Update tags" {
        n138 = Variant To Data(error in=w492, type=w497, Variant=w498) -> (data=w499:T2, error out=w500:errorcluster)
        n139 = Select(t=w497, s=w500, f=w499) -> (s? t:f=w496:T2)
        n140 = case shown="\"Waiting for Stop (Acq Stopped)\"" w488 {
          tunnel: w492 -> [w502 w506]
          tunnel: w491 -> [_ w505]
          tunnel: [w502 w504] -> w490
          frame "Idle", Default {
          }
          frame "Waiting for Stop (Acq Stopped)" {
            n141 = call-poly "Enqueue Message.vi"("error in (no error)"=w506, "Message"="Acq report", "Message Queue"=w505) -> ("error out"=w504:errorcluster)  [unwired: 7 in, 1 out]
          }
        }
      }
      frame "Acq report" {
        n142 = Unbundle By Name(w522) -> ("TAGs"=w515:string[])
        n143 = Unbundle By Name(w523) -> ("FPGA error"=w521:errorcluster, "data"=w520:dbl[], "Direccion 0?"=w516:bool)
        n144 = Unbundle By Name(w519) -> ("File path.Reporting Adquisición"=w518:path)
        n145 = Bundle("FPGA error"=w521, "data"=w520, "TAGs"=w515, "Direccion 0?"=w516) -> (w517:T12)  [unwired: 1 in]
        n146 = call "Reporting_acq_inycom.vi"("input cluster"=w517, "address repoting"=w518) -> ("Reporting"=w512:string)  [unwired: 1 in]
        n147 = call-poly "Enqueue Message.vi"("error in (no error)"=w511, "Message Data"=w512, "Message"="Update Status", "Message Queue"=w514) -> ("error out"=w509:errorcluster, "dup Message Queue"=w510:refnum<queue>)  [unwired: 6 in]
        n148 = call-poly "Enqueue Message.vi"("error in (no error)"=w509, "Message"="Exit Acq", "Message Queue"=w510) -> ("error out"=w508:errorcluster)  [unwired: 7 in, 1 out]
      }
      frame "Exit Acq" {
        n149 = Unbundle By Name(w532) -> ("FPGA error.status"=w540:bool, "File error.status"=w539:bool, "FPGA error"=w530:errorcluster, "File error"=w531:errorcluster)
        n150 = Unbundle By Name(w542) -> ("Timeout ruedas"=w533:bool)
        n151 = Merge Errors(w530, w531) -> (w528:errorcluster)
        n152 = Compound Arithmetic op=OR(w533, w540, w539) -> (w529:bool)
        n153 = case shown="False" w529 {
          tunnel: w541 -> [w548 w555]
          tunnel: [w550 w554] -> w536
          tunnel: w527 -> [w549 w553]
          tunnel: w528 -> [_ w551]
          frame False {
            n154 = call-poly "Enqueue Message.vi"("error in (no error)"=w549, "Message"="Procesado", "Message Queue"=w548) -> ("error out"=w550:errorcluster)  [unwired: 7 in, 1 out]
          }
          frame True {
            n155 = call-poly "Enqueue Message.vi"("error in (no error)"=w553, "Message Data"=w551, "Message"="Test" ("t"), "Message Queue"=w555) -> ("error out"=w554:errorcluster)  [unwired: 6 in, 1 out]
          }
        }
        n156 = call-poly "Enqueue Message.vi"("error in (no error)"=w527, "Message"="Clear", "Message Queue"=w534) -> ("error out"=w537:errorcluster)  [unwired: 7 in, 1 out]
        n157 = Merge Errors(w537, w536) -> (w535:errorcluster)
      }
      frame "Procesado" {
        n158 = call "Reporting_datetime.vi"() -> ("String"=w570:string)  [unwired: 11 in]
        n159 = Concatenate Strings(w570, "\nSTATUS: PROCESSING\nProcessing the measurement\n\n") -> (w565:string)
        n160 = call-poly "Enqueue Message.vi"("error in (no error)"=w557, "Message"="Start", "Message Queue"=w558) -> ("error out"=w561:errorcluster)  [unwired: 7 in, 1 out]
        n161 = call-poly "Enqueue Message.vi"("error in (no error)"=w557, "Message Data"=300.0, "Message"="Configuration", "Message Queue"=w563) -> ("error out"=w562:errorcluster)  [unwired: 6 in, 1 out]
        n162 = call-poly "Enqueue Message.vi"("error in (no error)"=w557, "Message Data"=w565, "Message"="Update Status", "Message Queue"=w566) -> ("error out"=w560:errorcluster)  [unwired: 6 in, 1 out]
        n163 = Merge Errors(w562, w561, w560) -> (w559:errorcluster)
      }
      frame "Update AURA" {
        n164 = Unbundle By Name(w579) -> ("Cfg.Report_AURA"=w581:string)
        n165 = Variant To Data(error in=w582, type=w581, Variant=w580) -> (data=w583:string, error out=w584:errorcluster)
        n166 = Select(t=w581, s=w584, f=w583) -> (s? t:f=w577:string)
        n167 = Bundle By Name(cluster=w579, "Cfg.Report_AURA"=w577) -> (w578:cluster{"File path":T5, "Cfg ":T7})
      }
      frame "Error" {
        # "Error - Display an error dialog. This message is sent by the \"Error Handler\" VIs at the end of other loops in this application."
        n168 = Variant To Data(error in=w595, type=errorcluster {"status"=FALSE, "code"=0, "source"=""} ("error constant"), Variant=w598) -> (data=→"error":errorcluster, error out=w599:errorcluster)
        n169 = Merge Errors(w599) -> (w597:errorcluster)
      }
      frame "Confirm Quit" {
        # "Confirm Quit - Message that can confirm whether or not the user wants to exit the application."
        n170 = case shown="\"Acquiring and Logging\"" w610 {
          tunnel: w609 -> [w617 w621]
          tunnel: w608 -> [w616 w620]
          tunnel: [w615 w619] -> w607
          tunnel: [UI_State."Idle" ("UI State") w618] -> w606
          frame Default {
            # "If 'Confirm Quit' comes in while the system is idle, there is no need for a confirmation message."
            n171 = call-poly "Enqueue Message.vi"("Priority Message? (F)"=TRUE, "error in (no error)"=w616, "Message"="Exit", "Message Queue"=w617) -> ("error out"=w615:errorcluster)  [unwired: 6 in, 1 out]
          }
          frame "Acquiring and Logging" {
            n172 = Two Button Dialog(message="Are you sure you want to quit while the acquisition is running?" ("Confirm Quit Message"), 1:"No" ("No"), 2:"Yes" ("Yes")) -> (T button?=w622:bool)
            n173 = case shown="True" w622 {
              tunnel: w621 -> [_ w631]
              tunnel: w620 -> [w627 w632]
              tunnel: [w627 w630] -> w619
              tunnel: [UI_State."Acquiring and Logging" ("UI State") UI_State."Waiting for Exit" ("UI State")] -> w618
              frame False {
                # "User did not want to quit."
              }
              frame True {
                n174 = call-poly "Enqueue Message.vi"("error in (no error)"=w632, "Message"="Stop", "Message Queue"=w631) -> ("error out"=w630:errorcluster)  [unwired: 7 in, 1 out]
              }
            }
          }
        }
      }
      frame "Exit" {
        # "Stop the VI"
        # "Exit - Send Exit messages to the Acquisition and Logging loops, and fire the user event to stop the Event Handling Loop."
        n175 = Variant To Data(type=errorcluster {"status"=FALSE, "code"=0, "source"=""} ("error constant"), Variant=w642) -> ()  [unwired: 1 in, 2 out]
        n176 = call <vilib>:"Simple Error Handler.vi"() -> ()  [unwired: 5 in, 5 out]
        n177 = call "close references.vi"("Watchdog"=w638, "Calibration"=w633, "Processing"=w639, "Acquisition"=w640, "RFID"=w646, "error in (no error)"=w644) -> ("error out"=w637:errorcluster)  [unwired: 9 in]
        n178 = call "Fire User Event - Stop.vi"("error in (no error)"=w637, "User Event - Stop"=w649) -> ("error out"=w648:errorcluster)  [unwired: 9 in]
      }
      frame "---Copy This Frame---" {
        # "Duplicate this frame when creating new messages.  Change this comment in the duplicated frame to describe this message."
        n179 = Merge Errors(w658) -> (w657:errorcluster)
      }
      frame Default {
        # "'Default' case only runs if there is a message that isn't defined in any of the other cases.  Output a programming error."
        n180 = xnode "Error Ring"("parameter 0"=w664) -> ("error out"=w663:errorcluster)
      }
    }
    n181 = call "Error Handler - Message Handling Loop.vi"("error in (no error)"=w48, "Message Queue"=w47) -> ("dup error in"=w49:errorcluster)  [unwired: 8 in, 1 out]
  }
  n182 = while {
    tunnel: w25 -> [w679]
    tunnel: [w676] -> w32
    shift-right: [w678] -> w30
    shift-left: w24 -> [w680]
    stop <- w677 stop-if-true
    # "Event Handling Loop"
    n183 = event shown="[3] \"Calibration\": Value Change" {
      selector: w680 -> [_ _ _ _ _ _]
      dyn-events: [_ _ _ _ _ _] -> w678
      timeout: _ -> [_ _ _ _ _ _]
      tunnel: [_ _ _ _ _ TRUE ("Discard?")] -> w677
      tunnel: w679 -> [w684 w687 w689 w696 w700 w704]
      tunnel: [w682 _ w692 w694 w699 _] -> w675
      tunnel: [w683 w687 w688 w695 w698 w704] -> w674
      event Panel Close? {
        # "Send the 'Confirm Quit' message if the user closes the panel of the VI. Discard the event so the 'Confirm Quit' message has a chance to run."
        n184 = event-data() -> ()  [unwired: 1 in, 1 out]
        n185 = call-poly "Enqueue Message.vi"("Priority Message? (F)"=TRUE, "Message"="Confirm Quit", "Message Queue"=w684) -> ("error out"=w682:errorcluster, "dup Message Queue"=w683:refnum<queue>)  [unwired: 7 in]
        n186 = event-data("Discard?"=TRUE) -> ()  [unwired: 1 in, 1 out]
      }
      event Application Instance Close {
        n187 = event-data() -> ()  [unwired: 1 in, 1 out]
      }
      event "Exit": Value Change {
        w690 = TRUE  # Priority Message
        # "The UI Message Loop handles sending the Exit message to other loops."
        n188 = event-data() -> ()  [unwired: 1 in, 1 out]
        n189 = call-poly "Enqueue Message.vi"("Priority Message? (F)"=w690, "Message"="Exit", "Message Queue"=w689) -> ("error out"=w692:errorcluster, "dup Message Queue"=w688:refnum<queue>)  [unwired: 7 in]
      }
      event "Calibration": Value Change {
        n190 = event-data() -> ()  [unwired: 1 in, 1 out]
        n191 = call-poly "Enqueue Message.vi"("Message"="Calibration", "Message Queue"=w696) -> ("error out"=w694:errorcluster, "dup Message Queue"=w695:refnum<queue>)  [unwired: 8 in]
      }
      event "Developer commad": Value Change {
        n192 = event-data() -> ("NewVal"=w697:string)  [unwired: 1 in]
        n193 = call-poly "Enqueue Message.vi"("Message"=w697, "Message Queue"=w700) -> ("error out"=w699:errorcluster, "dup Message Queue"=w698:refnum<queue>)  [unwired: 8 in]
      }
      event User Event {
        # "The Message Handling Loop processed an \"Exit\" message, which fired this event to stop the Event Handling Loop."
        n194 = event-data() -> ()  [unwired: 1 in, 1 out]
        n195 = local read "Report"() -> (w701:string)
        n196 = Concatenate Strings("Exit" ("Exit String"), w701) -> (w703:string)
        n197 = local write "Report"(w703) -> ()
      }
    }
    n198 = call "Error Handler - Event Handling Loop.vi"("error in (no error)"=w675, "Message Queue"=w674) -> ("dup error in"=w676:errorcluster)  [unwired: 8 in, 1 out]
  }
  n199 = Unregister For Events(event registration refnum=w30, error in=w32) -> (error out=w31:errorcluster)
  n200 = Release Queue(queue=w25, error in (no error)=w33) -> (error out=w20:errorcluster)  [unwired: 1 in, 2 out]
  n201 = Merge Errors(w31, w20) -> (w26:errorcluster)
  n202 = call "Destroy User Event - Stop.vi"("error in (no error)"=w26, "User Event - Stop"=w23) -> ()  [unwired: 9 in, 1 out]
